vi "stop-start_Control.vi"(8 "error in (no error)":errorcluster, 11 "Automation Refnum in":refnum<k7>) -> (0 "error out":errorcluster, 3 "Automation Refnum out":refnum<k7>)   [LabVIEW 2021]
doc: "André Romero - 2024\nandretec@ifsc.usp.br\nIFSC - USP"
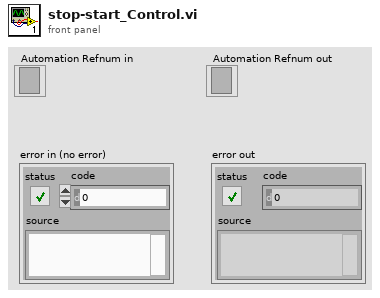
[diagram p1: front panel]
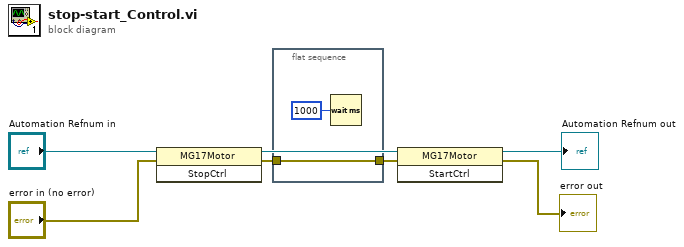
[diagram p0: block diagram]
diagram:
  n1 = invoke class="MG17Motor" method="StopCtrl"(reference="Automation Refnum in", error in="error in (no error)") -> (reference out=w5:refnum<k7>, error out=w2:errorcluster)  [unwired: 1 in, 1 out]
  n2 = flat-sequence {
    tunnel: w2 -> [w9]
    tunnel: [w9] -> w1
    frame #0 {
      n3 = Wait (ms)(milliseconds to wait=u32 1000) -> ()  [unwired: 1 out]
    }
  }
  n4 = invoke class="MG17Motor" method="StartCtrl"(reference=w5, error in=w1) -> (reference out=→"Automation Refnum out":refnum<k7>, error out=→"error out":errorcluster)  [unwired: 1 in, 1 out]
